vi "Test LGP5 Acquisition API.vi"() -> ()   [LabVIEW 2018]
doc: "LGP5 Acquisition API Tester."
uses:
  LGP5 Acquisition.lvlib
panel:
  out "HW ID":string
  in  "Test Start Acquiring":bool
  in  "Run as Singleton?":bool
  in  "Show Block Diagram":bool
  in  "Refresh Modules":bool
  out "Active Modules":string[](array[string])
  in  "Stop Module":bool
  in  "Select Module":i32(ring)=-1 caption="Select Module\nTo send Request to" items=["All"=-1, "4140002"=4140002, "4140003"=4140003]
  in  "Run New Module":bool
  in  "Hide Module Panel":bool
  in  "Show Module Panel":bool
  out "Status":string
  # "This VI tests the API for the Module."
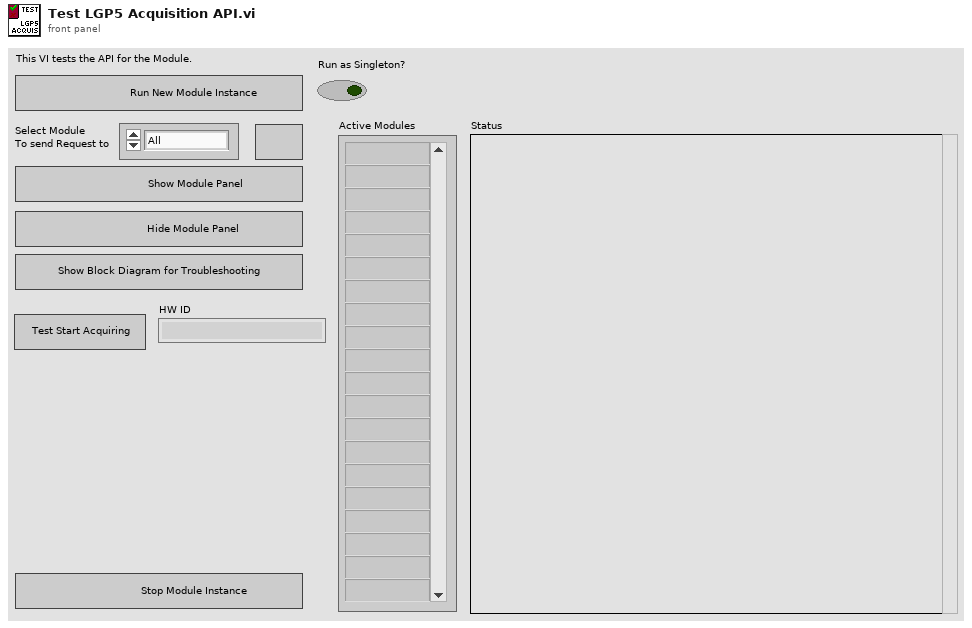
[diagram p1: front panel]
types:
  T1 = typedef "LGP5 Acquisition.lvlib/Broadcast Events--cluster.ctl" = cluster{"Module Did Init":refnum<user-event>, "Status Updated":refnum<user-event>, "Error Reported":refnum<user-event>, "Module Did Stop":refnum<user-event>, "Update Module Execution Status":refnum<user-event>, "Acquisition Started":refnum<user-event>}
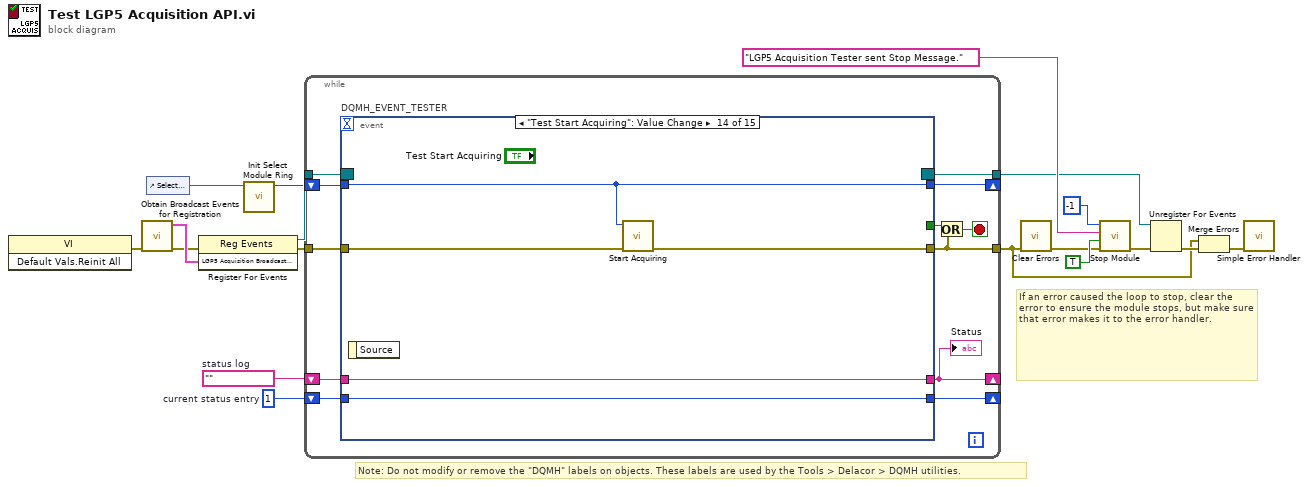
[diagram p0: block diagram]
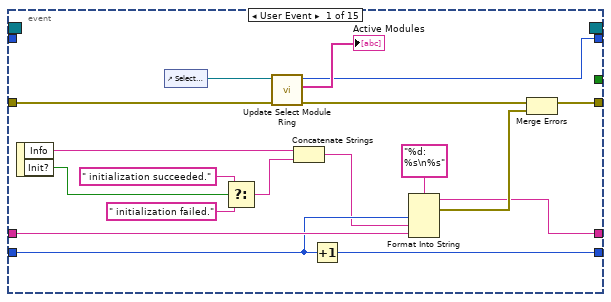
[diagram p2: hidden frame]
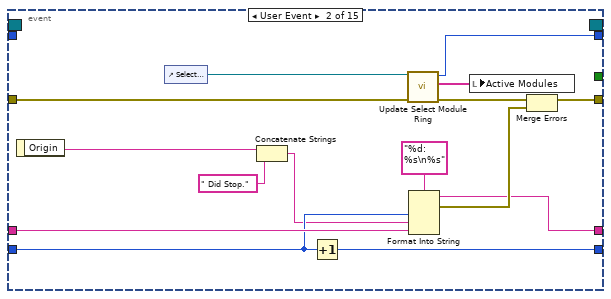
[diagram p3: hidden frame]
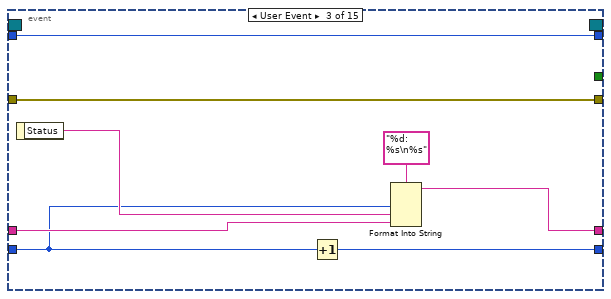
[diagram p4: hidden frame]
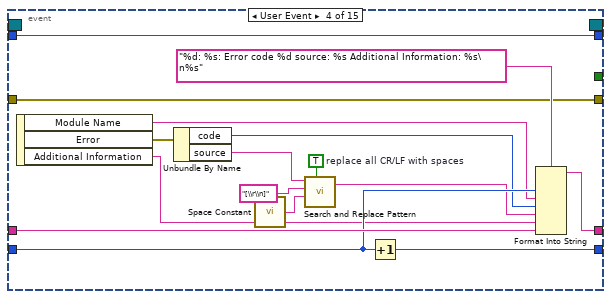
[diagram p5: hidden frame]
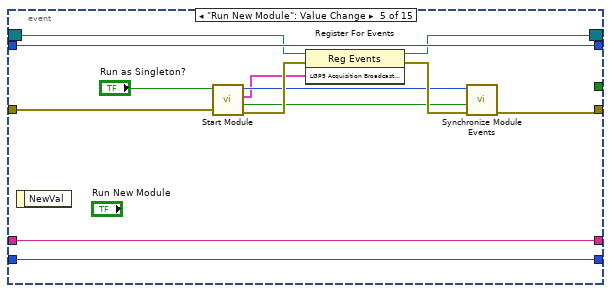
[diagram p6: hidden frame]
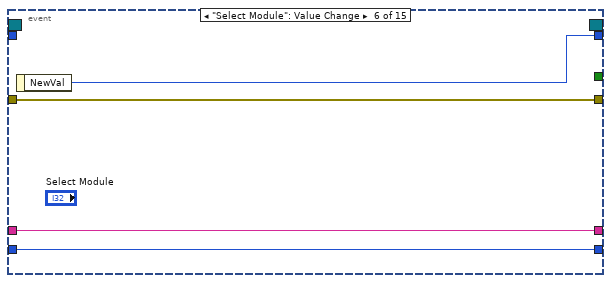
[diagram p7: hidden frame]
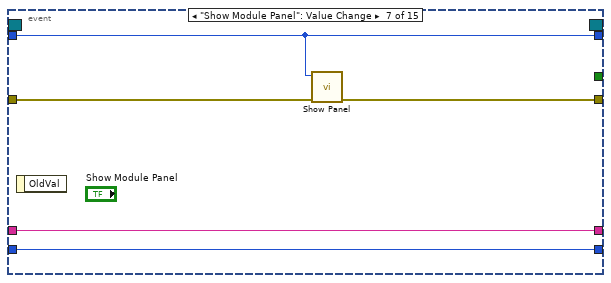
[diagram p8: hidden frame]
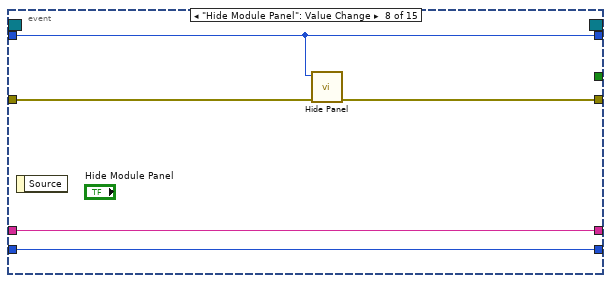
[diagram p9: hidden frame]
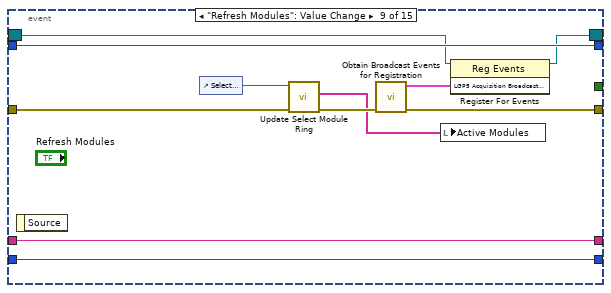
[diagram p10: hidden frame]
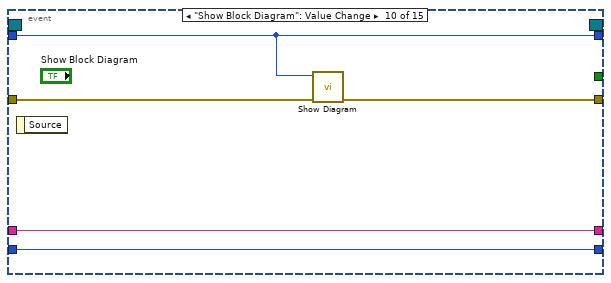
[diagram p11: hidden frame]
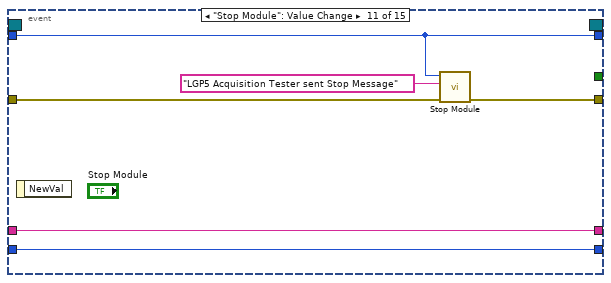
[diagram p12: hidden frame]
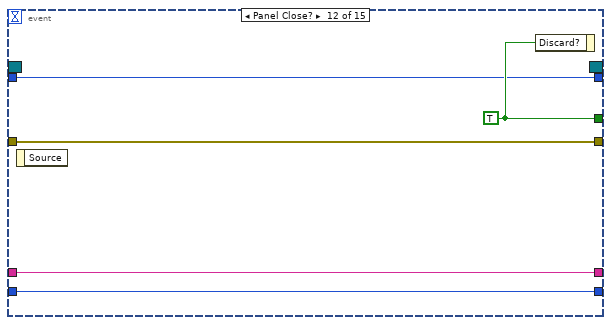
[diagram p13: hidden frame]
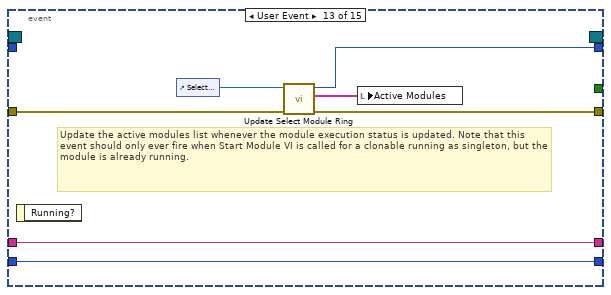
[diagram p14: hidden frame]
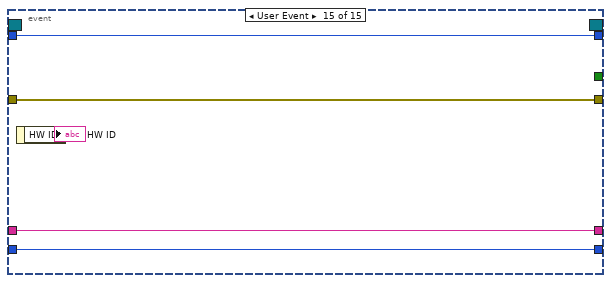
[diagram p15: hidden frame]
diagram:
  w14 = 1  # current status entry
  w15 = ""  # status log
  # "If an error caused the loop to stop, clear the error to ensure the module stops, but make sure that error makes it to the error handler."
  # "Note: Do not modify or remove the \"DQMH\" labels on objects. These labels are used by the Tools > Delacor > DQMH utilities."
  n1 = invoke class="VI" method="Default Vals.Reinit All"() -> (error out=w2:errorcluster)  [unwired: 3 in, 2 out]
  n2 = call "Obtain Broadcast Events for Registration.vi"("error in (no error)"=w2) -> ("error out"=w1:errorcluster, "LGP5 Acquisition Broadcast Events"=w11:T1)  [unwired: 9 in]
  n3 = control-ref of="Select Module"() -> (w12:refnum<vi>)
  n4 = register-events(error in=w1, w11) -> (reference out=w18:refnum<event-registration>, error out=w10:errorcluster)  [unwired: 1 in]
  n5 = call "Init Select Module Ring.vi"("Select Module Ring Ref"=w12) -> ("Value for All Modules"=w13:i32)  [unwired: 8 in, 2 out]
  n6 = while {
    tunnel: w18 -> [w30]
    tunnel: [w19] -> w3
    tunnel: w10 -> [w28]
    shift-right: [w24] -> _
    shift-left: w15 -> [w26]
    shift-right: [w25] -> _
    shift-left: w14 -> [w27]
    shift-right: [w21] -> _
    shift-left: w13 -> [w22]
    tunnel: [w20] -> w7
    stop <- w23 stop-if-true
    n7 = event "DQMH_EVENT_TESTER" shown="[13] \"Test Start Acquiring\": Value Change" {
      selector: w30 -> [_ _ _ _ w94 _ _ _ w120 _ _ _ _ _ _]
      dyn-events: [_ _ _ _ w93 _ _ _ w119 _ _ _ _ _ _] -> w20
      timeout: _ -> [_ _ _ _ _ _ _ _ _ _ _ _ _ _ _]
      tunnel: [_ _ _ _ _ _ _ _ _ _ _ w141 _ _ _] -> w29
      tunnel: [w38 w55 w71 w77 w92 w104 w108 w113 w116 w127 w132 w140 w144 w150 w158] -> w19
      tunnel: w28 -> [w40 w57 w71 w77 w95 w104 w109 w114 w121 w130 w133 w140 w145 w153 w158]
      tunnel: w27 -> [w45 w60 w64 w83 w97 w102 w106 w111 w124 w128 w135 w138 w147 w151 w156]
      tunnel: w26 -> [w46 w61 w67 w85 w98 w103 w107 w112 w125 w129 w136 w139 w148 w152 w157]
      tunnel: [w43 w58 w68 w80 w98 w103 w107 w112 w125 w129 w136 w139 w148 w152 w157] -> w24
      tunnel: [w44 w59 w70 w86 w97 w102 w106 w111 w124 w128 w135 w138 w147 w151 w156] -> w25
      tunnel: w22 -> [_ _ w65 w87 w96 _ w105 w110 w123 w126 w134 w137 _ w149 w155]
      tunnel: [w35 w52 w65 w87 w96 w101 w105 w110 w123 w126 w134 w137 w143 w149 w155] -> w21
      event User Event {
        n8 = event-data() -> ("Info"=w42:string, "Init?"=w32:bool)  [unwired: 1 in]
        n9 = control-ref of="Select Module"() -> (w37:refnum<vi>)
        n10 = Select(t=" initialization succeeded.", s=w32, f=" initialization failed.") -> (s? t:f=w31:string)
        n11 = call "Update Select Module Ring.vi"("error in (no error)"=w40, "Select Module Ring Ref"=w37) -> ("error out"=w39:errorcluster, "Active Modules (Array)"=→"Active Modules":string[], "New Module Ring Value"=w35:i32)  [unwired: 7 in]
        n12 = Concatenate Strings(w42, w31) -> (w41:string)
        n13 = Increment(x=w45) -> (x+1=w44:i32)
        n14 = Format Into String(format string="%d: %s\n%s", w45, w41, w46) -> (resulting string=w43:string, error out=w48:errorcluster)  [unwired: 2 in]
        n15 = Merge Errors(w39, w48) -> (w38:errorcluster)
      }
      event User Event {
        n16 = event-data() -> ("Origin"=w50:string)  [unwired: 1 in]
        n17 = control-ref of="Select Module"() -> (w54:refnum<vi>)
        n18 = Concatenate Strings(w50, " Did Stop.") -> (w49:string)
        n19 = Increment(x=w60) -> (x+1=w59:i32)
        n20 = call "Update Select Module Ring.vi"("error in (no error)"=w57, "Select Module Ring Ref"=w54) -> ("error out"=w56:errorcluster, "Active Modules (Array)"=w53:string[], "New Module Ring Value"=w52:i32)  [unwired: 7 in]
        n21 = Format Into String(format string="%d: %s\n%s", w60, w49, w61) -> (resulting string=w58:string, error out=w63:errorcluster)  [unwired: 2 in]
        n22 = local write "Active Modules"(w53) -> ()
        n23 = Merge Errors(w56, w63) -> (w55:errorcluster)
      }
      event User Event {
        n24 = event-data() -> ("Status"=w66:string)  [unwired: 1 in]
        n25 = Increment(x=w64) -> (x+1=w70:i32)
        n26 = Format Into String(format string="%d: %s\n%s", w64, w66, w67) -> (resulting string=w68:string)  [unwired: 2 in, 1 out]
      }
      event User Event {
        w81 = TRUE  # replace all CR/LF with spaces
        n27 = event-data() -> ("Module Name"=w75:string, "Error"=w74:errorcluster, "Additional Information"=w72:string)  [unwired: 1 in]
        n28 = Unbundle By Name(w74) -> ("code"=w76:i32, "source"=w78:string)
        n29 = call <vilib>:"Space Constant.vi"() -> ("String"=w82:string)
        n30 = call <vilib>:"Search and Replace Pattern.vi"("string"=w78, "regular expression (\"\")"="[\\r\\n]" ("regular expression (\"\")"), "replace string (\"\")"=w82, "replace all? (F)"=w81) -> ("result string"=w79:string)  [unwired: 1 in, 1 out]
        n31 = Increment(x=w83) -> (x+1=w86:i32)
        n32 = Format Into String(format string="%d: %s: Error code %d source: %s Additional Information: %s\n%s", w83, w75, w76, w79, w72, w85) -> (resulting string=w80:string)  [unwired: 2 in, 1 out]
      }
      event "Run New Module": Value Change {
        n33 = event-data() -> ()  [unwired: 1 in, 1 out]
        n34 = call "Start Module.vi"("error in (no error)"=w95, "Run as Singleton? (F)"="Run as Singleton?") -> ("error out"=w99:errorcluster, "Wait for Event Sync?"=w90:bool, "LGP5 Acquisition Broadcast Events"=w89:T1, "Module ID"=w91:i32)  [unwired: 6 in]
        n35 = register-events(reference=w94, error in=w99, w89) -> (reference out=w93:refnum<event-registration>, error out=w100:errorcluster)
        n36 = call "Synchronize Module Events.vi"("error in (no error)"=w100, "Wait for Event Sync?"=w90, "Module ID"=w91) -> ("error out"=w92:errorcluster)  [unwired: 7 in, 1 out]
      }
      event "Select Module": Value Change {
        n37 = event-data() -> ("NewVal"=w101:i32)  [unwired: 1 in]
      }
      event "Show Module Panel": Value Change {
        n38 = event-data() -> ()  [unwired: 1 in, 1 out]
        n39 = call "Show Panel.vi"("error in (no error)"=w109, "Module ID"=w105) -> ("error out"=w108:errorcluster)  [unwired: 9 in]
      }
      event "Hide Module Panel": Value Change {
        n40 = event-data() -> ()  [unwired: 1 in, 1 out]
        n41 = call "Hide Panel.vi"("error in (no error)"=w114, "Module ID"=w110) -> ("error out"=w113:errorcluster)  [unwired: 9 in]
      }
      event "Refresh Modules": Value Change {
        n42 = event-data() -> ()  [unwired: 1 in, 1 out]
        n43 = control-ref of="Select Module"() -> (w122:refnum<vi>)
        n44 = call "Update Select Module Ring.vi"("error in (no error)"=w121, "Select Module Ring Ref"=w122) -> ("error out"=w117:errorcluster, "Active Modules (Array)"=w115:string[])  [unwired: 7 in, 1 out]
        n45 = call "Obtain Broadcast Events for Registration.vi"("error in (no error)"=w117) -> ("error out"=w116:errorcluster, "LGP5 Acquisition Broadcast Events"=w118:T1)  [unwired: 9 in]
        n46 = local write "Active Modules"(w115) -> ()
        n47 = register-events(reference=w120, w118) -> (reference out=w119:refnum<event-registration>)  [unwired: 1 in, 1 out]
      }
      event "Show Block Diagram": Value Change {
        n48 = event-data() -> ()  [unwired: 1 in, 1 out]
        n49 = call "Show Diagram.vi"("error in (no error)"=w130, "Module ID"=w126) -> ("error out"=w127:errorcluster)  [unwired: 9 in]
      }
      event "Stop Module": Value Change {
        n50 = event-data() -> ()  [unwired: 1 in, 1 out]
        n51 = call "Stop Module.vi"("error in (no error)"=w133, "Origin"="LGP5 Acquisition Tester sent Stop Message", "Module ID"=w134) -> ("error out"=w132:errorcluster)  [unwired: 8 in]
      }
      event Panel Close? {
        w141 = TRUE ("Discard?")
        n52 = event-data() -> ()  [unwired: 1 in, 1 out]
        n53 = event-data("Discard?"=w141) -> ()  [unwired: 1 in, 1 out]
      }
      event User Event {
        # "Update the active modules list whenever the module execution status is updated. Note that this event should only ever fire when Start Module VI is called for a clonable running as singleton, but the module is already running."
        n54 = event-data() -> ()  [unwired: 1 in, 1 out]
        n55 = control-ref of="Select Module"() -> (w146:refnum<vi>)
        n56 = call "Update Select Module Ring.vi"("error in (no error)"=w145, "Select Module Ring Ref"=w146) -> ("error out"=w144:errorcluster, "Active Modules (Array)"=w142:string[], "New Module Ring Value"=w143:i32)  [unwired: 7 in]
        n57 = local write "Active Modules"(w142) -> ()
      }
      event "Test Start Acquiring": Value Change {
        n58 = event-data() -> ()  [unwired: 1 in, 1 out]
        n59 = call "Start Acquiring.vi"("error in (no error)"=w153, "Module ID"=w149) -> ("error out"=w150:errorcluster)  [unwired: 7 in, 2 out]
      }
      event User Event {
        n60 = event-data() -> ("HW ID"=→"HW ID":string)  [unwired: 1 in]
      }
    }
    "Status" <- w24
    n61 = Or(x=w29, y=w19) -> (x .or. y?=w23:bool)
  }
  n62 = call <vilib>:"Clear Errors.vi"("error in (no error)"=w3) -> ("error out"=w5:errorcluster)  [unwired: 5 in, 1 out]
  n63 = call "Stop Module.vi"("error in (no error)"=w5, "Wait for Module to stop? (F)"=TRUE ("Wait for Module to stop?"), "Origin"="LGP5 Acquisition Tester sent Stop Message.", "Module ID"=-1 ("Stop all")) -> ("error out"=w16:errorcluster)  [unwired: 7 in]
  n64 = Unregister For Events(event registration refnum=w7, error in=w16) -> (error out=w17:errorcluster)
  n65 = Merge Errors(w3, w17) -> (w4:errorcluster)
  n66 = call <vilib>:"Simple Error Handler.vi"("error in (no error)"=w4) -> ()  [unwired: 4 in, 5 out]
